vi "Example_DataRecording.vi"() -> ()   [LabVIEW 2018]
doc: "Example how to configure and use the data recording functions. Before starts this example the device must be tuned and the parameter settings must be correct.\nThe example shows:\n - how to initialise and close an interface (e.g. RS232)\n - configuration of the data recorder\n - start of a relative positioning\n - show the recorded data (position, velocity and current)"
panel:
  out "Current Graph":i16[](graph)
  out "Velocity Graph":i32[](graph)
  out "Position  Graph":i32[](graph)
  in  "timeout":u32=1000
  in  "relative position":i32=100
  in  "position profile":T1={"profileVelocity"=1000, "profileAcceleration"=10000, "profileDeceleration"=10000}
  in  "nodeId":u16=1
  in  "communication settings in":T2={"deviceName"="EPOS2", "protocolStackName"="MAXON SERIAL V2", "interfaceName"="USB", "portName"="USB0", "baudrate"=1000000, "timeout"=500}
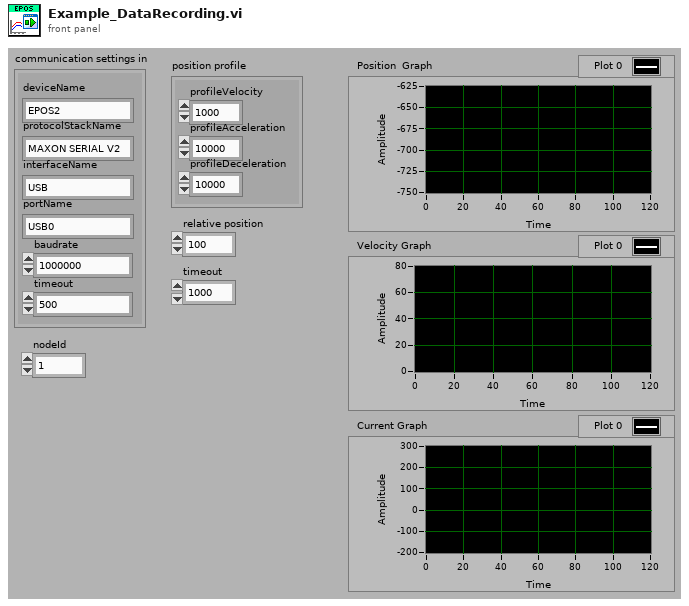
[diagram p1: front panel]
types:
  T1 = cluster{"profileVelocity":u32, "profileAcceleration":u32, "profileDeceleration":u32}
  T2 = cluster{"deviceName":string, "protocolStackName":string, "interfaceName":string, "portName":string, "baudrate":u32, "timeout":u32}
  T3 = cluster{"recorded object 1":cluster{"objectIndex":u16, "objectSubIndex":u8, "objectSize":u8}, "recorded object 2":cluster{"objectIndex":u16, "objectSubIndex":u8, "objectSize":u8}, "recorded object 3":cluster{"objectIndex":u16, "objectSubIndex":u8, "objectSize":u8}, "recorded object 4":cluster{"objectIndex":u16, "objectSubIndex":u8, "objectSize":u8}}
  T4 = cluster{"samplingPeriod":u16, "nbOfPrecedingSamples":u16}
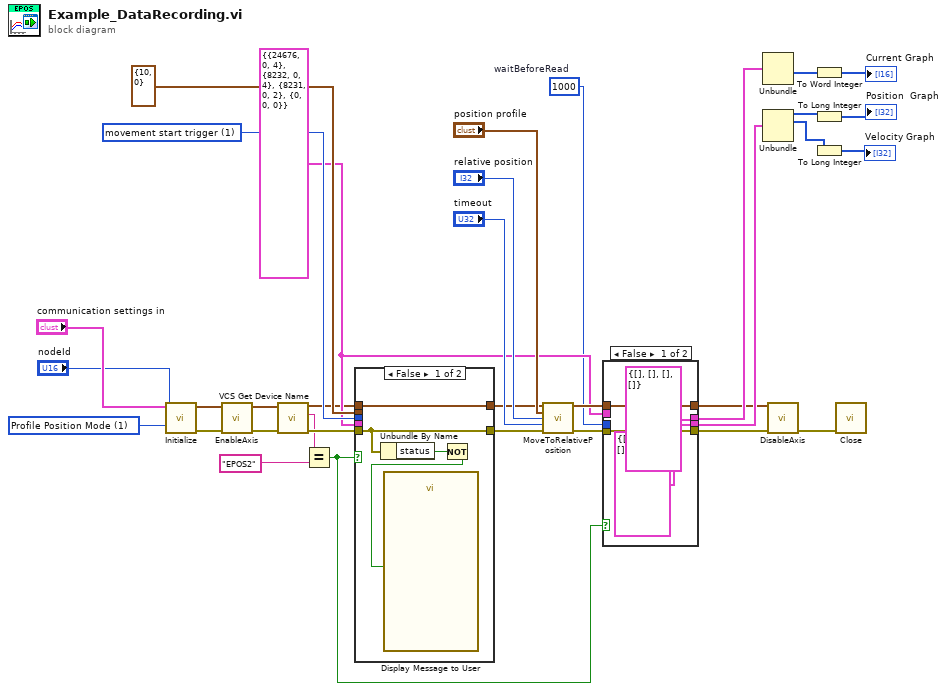
[diagram p0: block diagram]
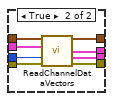
[diagram p2: hidden frame]
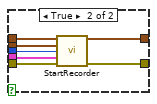
[diagram p3: hidden frame]
diagram:
  w19 = u32 1000  # waitBeforeRead
  w20 = T3 {"recorded object 1"={"objectIndex"=24676, "objectSubIndex"=0, "objectSize"=4}, "recorded object 2"={"objectIndex"=8232, "objectSubIndex"=0, "objectSize"=4}, "recorded object 3"={"objectIndex"=8231, "objectSubIndex"=0, "objectSize"=2}, "recorded object 4"={"objectIndex"=0, "objectSubIndex"=0, "objectSize"=0}} ("recorded objects")
  w25 = u8 1 items=["movement start trigger"=1, "error trigger"=2, "digital input trigger"=4, "movement end trigger"=8] ("trigger type")
  w33 = i8 1 items=["Profile Position Mode"=1, "Profile Velocity Mode"=3, "Homing Mode"=6, "Interpolated Position Mode"=7, "Position Mode"=-1, "Velocity Mode"=-2, "Current Mode"=-3, "Master Encoder Mode"=-5, "Step Direction Mode"=-6] ("modes of operations")
  n1 = call "Initialize.vi"("modes of operations"=w33, "nodeId"="nodeId", "communication settings in"="communication settings in") -> ("error out"=w31:errorcluster, "axis out"=w30:cluster{"keyHandle":u32, "nodeId":u16})  [unwired: 7 in]
  n2 = call "EnableAxis.vi"("error in (no error)"=w31, "axis in"=w30) -> ("error out"=w4:errorcluster, "axis out"=w5:cluster{"keyHandle":u32, "nodeId":u16})  [unwired: 4 in]
  n3 = call "VCS Get Device Name.vi"("error in (no error)"=w4, "axis in"=w5) -> ("error out"=w7:errorcluster, "deviceName"=w3:string, "axis out"=w6:cluster{"keyHandle":u32, "nodeId":u16})  [unwired: 7 in]
  n4 = Equal?(x=w3, y="EPOS2" ("x")) -> (x = y?=w1:bool)
  n5 = case shown="False" w1 {
    tunnel: T4 {"samplingPeriod"=10, "nbOfPrecedingSamples"=0} ("parameter") -> [_ w45]
    tunnel: w25 -> [_ w44]
    tunnel: [w37 w43] -> w24
    tunnel: [w38 w42] -> w23
    tunnel: w20 -> [_ w41]
    tunnel: w7 -> [w37 w40]
    tunnel: w6 -> [w38 w39]
    frame False {
      n6 = Unbundle By Name(w37) -> ("status"=w35:bool)
      n7 = Not(x=w35) -> (.not. x?=w36:bool)
      n8 = call "Display Message to User"("Enable"=w36) -> ()  [unwired: 9 in, 2 out]
    }
    frame True {
      n9 = call "StartRecorder.vi"("axis in"=w39, "parameter"=w45, "trigger type"=w44, "recorded objects"=w41, "error in (no error)"=w40) -> ("axis out"=w42:cluster{"keyHandle":u32, "nodeId":u16}, "error out"=w43:errorcluster)  [unwired: 9 in]
    }
  }
  n10 = call "MoveToRelativePosition.vi"("axis in"=w23, "position profile"="position profile", "relative position"="relative position", "timeout"="timeout", "error in (no error)"=w24) -> ("axis out"=w21:cluster{"keyHandle":u32, "nodeId":u16}, "error out"=w22:errorcluster)  [unwired: 9 in]
  n11 = case shown="False" w1 {
    tunnel: w22 -> [w48 w57]
    tunnel: w21 -> [w49 w56]
    tunnel: w20 -> [_ w55]
    tunnel: w19 -> [_ w54]
    tunnel: [cluster{u16[], u16[], u16[], u16[]} {[], [], [], []} ("U16 data vectors") w53] -> w18
    tunnel: [cluster{u32[], u32[], u32[], u32[]} {[], [], [], []} ("U32 data vectors") w52] -> w17
    tunnel: [w49 w51] -> w10
    tunnel: [w48 w50] -> w9
    frame False {
    }
    frame True {
      n12 = call "ReadChannelDataVectors.vi"("axis in"=w56, "recorded objects"=w55, "waitBeforeRead"=w54, "error in (no error)"=w57) -> ("axis out"=w51:cluster{"keyHandle":u32, "nodeId":u16}, "U16 data vectors"=w53:cluster{u16[], u16[], u16[], u16[]}, "U32 data vectors"=w52:cluster{u32[], u32[], u32[], u32[]}, "error out"=w50:errorcluster)  [unwired: 7 in, 1 out]
    }
  }
  n13 = Unbundle(w18) -> (w14:u16[])  [unwired: 3 out]
  n14 = Unbundle(w17) -> (w16:u32[], w15:u32[])  [unwired: 2 out]
  n15 = call "DisableAxis.vi"("error in (no error)"=w9, "axis in"=w10) -> ("error out"=w8:errorcluster)  [unwired: 4 in, 1 out]
  n16 = To Word Integer(number=w14) -> (16bit integer=→"Current Graph":i16[])
  n17 = To Long Integer(number=w16) -> (32bit integer=→"Position  Graph":i32[])
  n18 = To Long Integer(number=w15) -> (32bit integer=→"Velocity Graph":i32[])
  n19 = call "Close.vi"("error in (no error)"=w8) -> ()  [unwired: 10 in, 1 out]
